vi "Attributes Setup.vi"(11 "IMAQdx Cam in":refnum<class "IMAQdx Cam.lvclass">) -> ()   [LabVIEW 2020, in "IMAQdx Cam.lvclass"]
doc: "The Grab and Attributes Setup example VI allows the user to view the current attributes and settings, update attribute settings, acquire images continuously, and display the images in an image control."
uses:
  IMAQdx Cam.lvclass
  IMAQdx Cam.lvclass/IMAQdx Cam.ctl
panel:
  in  "Filter":string
  in  "error in":errorcluster
  out "Tooltip":string
  out "Units":string
  out "Tab Control Ref":T1
  in  "Tab Control":T2(tab)
  in  "U32 Value Control":u32(slide) scale=4.0..4044.0
  in  "DBL Value Control":dbl(slide) min=17.00000029813964 max=5000000.0 step=1.0 scale=17.00000029813964..5000000.0
  in  "String Value Control":string
  in  "Enum Value Control":u32(ring) items=["Use hardware value", "10-bit", "12-bit", "14-bit", "16-bit"]
  in  "Boolean Value Control":bool=TRUE
  in  "Command Value Control":bool
  in  "Attribute Table":string(tree)="_1"
  in  "stop":bool
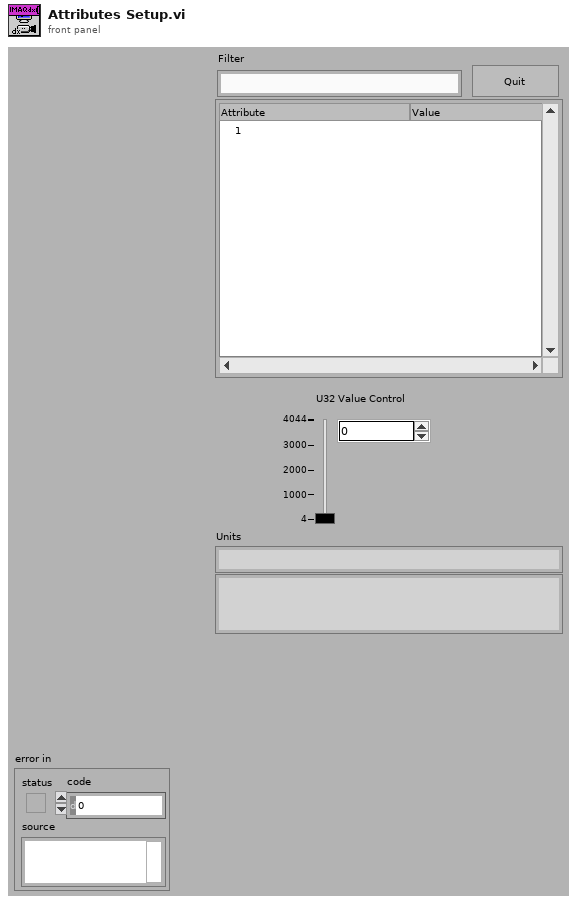
[diagram p1: front panel]
types:
  T1 = cluster{"Tab Control":refnum<vi>, "U32 Value Control":refnum<vi>, "DBL Value Control":refnum<vi>, "String Value Control":refnum<vi>, "Enum Value Control":refnum<vi>, "Boolean Value Control":refnum<vi>, "Command Value Control":refnum<vi>}
  T2 = enum32{"U32", "DBL", "String", "Enum", "Bool", "Command"}
  T3 = typedef "IMAQdx.ctl" = refnum<k21>
  T4 = typedef "eventvkey.ctl" = enum16{"ASCII", "Enter", "Return", "Shift", "Ctrl", "Alt", "Cmd", "Opt", "Caps", "NumLock", "Clear", "Break", "Up", "Down", "Left", "Right", "Insert", "Delete", "Home", "End", "PageUp", "PageDown", "Escape", "Help", "Pause", "ScrollLock", "F1", "F2", "F3", "F4", "F5", "F6", "F7", "F8", "F9", "F10", "F11", "F12", "F13", "F14", "F15", "F16", "F17", "F18", "F19", "F20", "F21", "F22", "F23", "F24", "Play", "VolumeUp", "VolumeDown", "Mute", "Two Byte Char"}
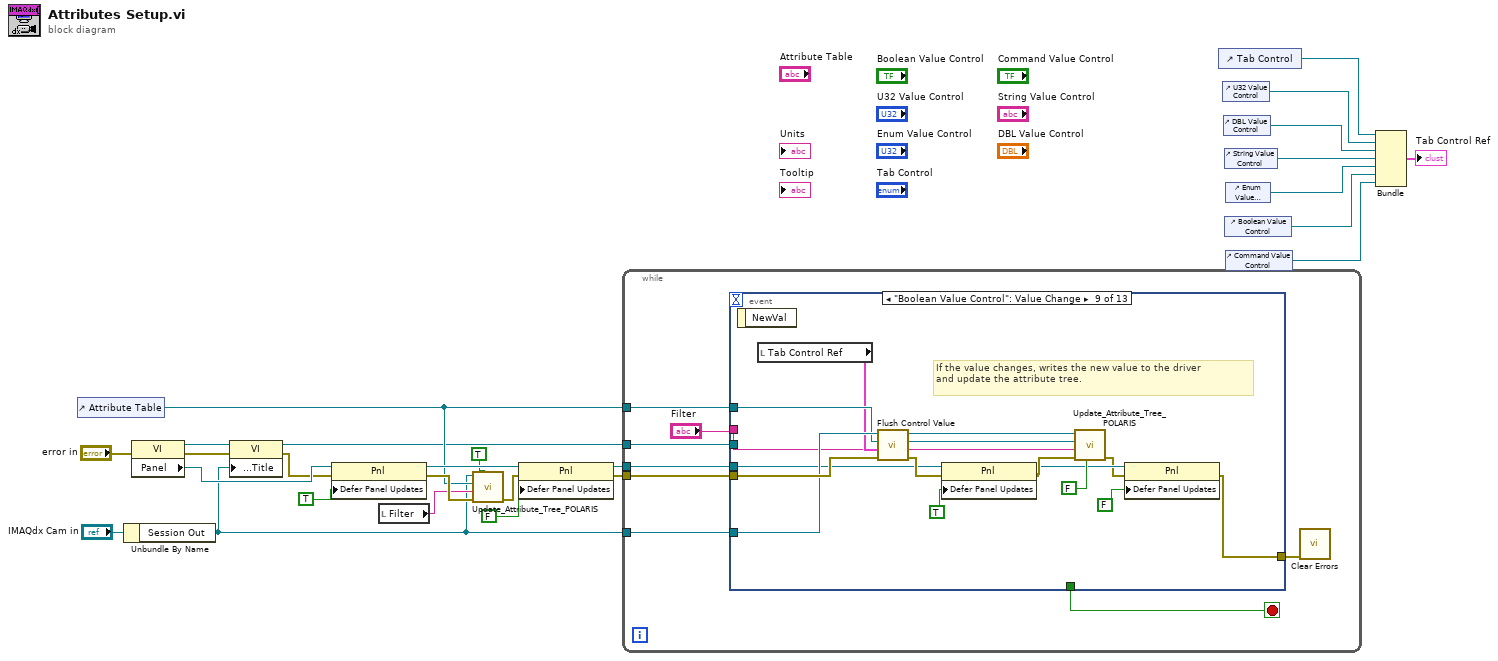
[diagram p0: block diagram]
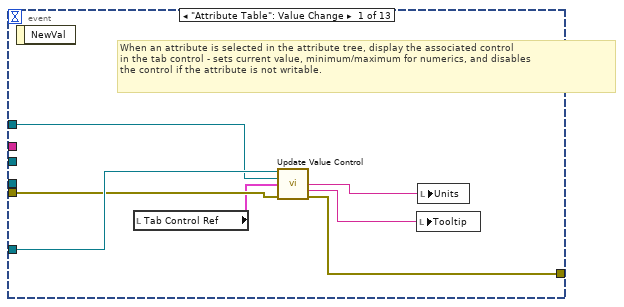
[diagram p2: hidden frame]
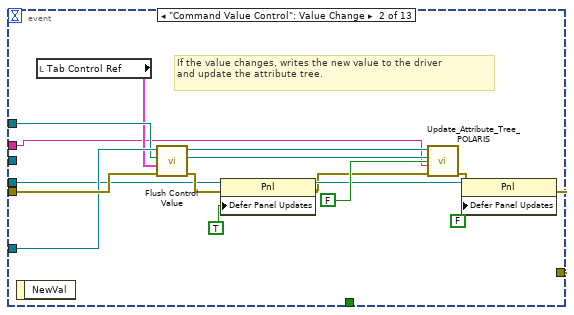
[diagram p3: hidden frame]
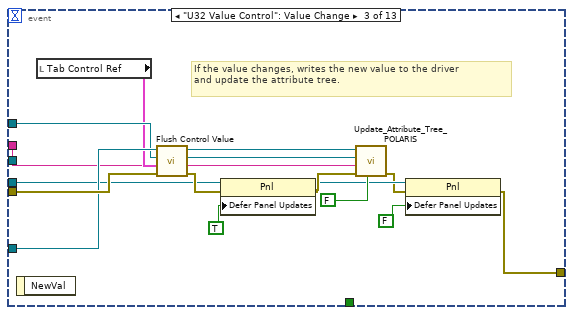
[diagram p4: hidden frame]
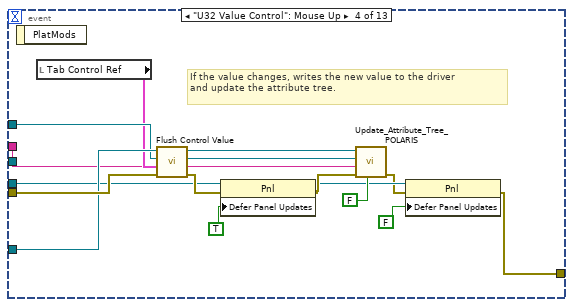
[diagram p5: hidden frame]
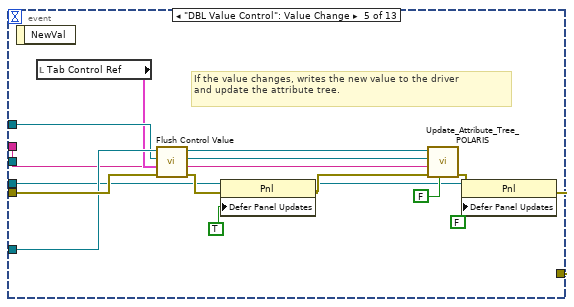
[diagram p6: hidden frame]
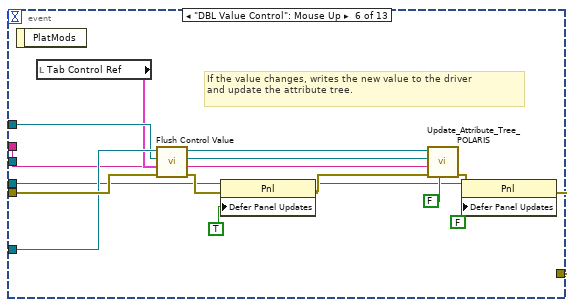
[diagram p7: hidden frame]
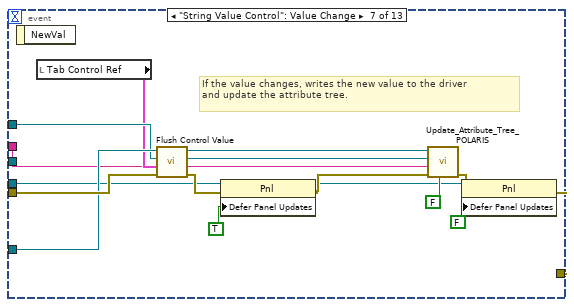
[diagram p8: hidden frame]
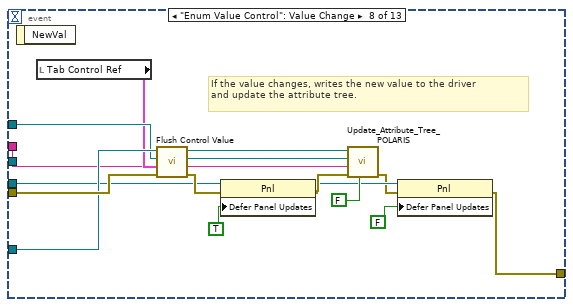
[diagram p9: hidden frame]
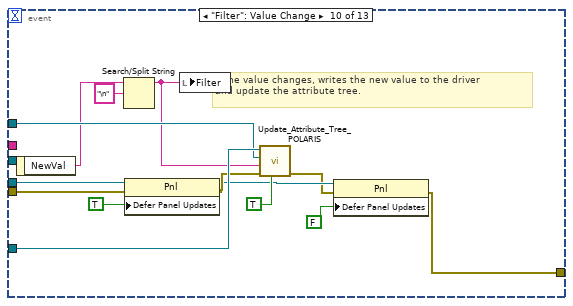
[diagram p10: hidden frame]
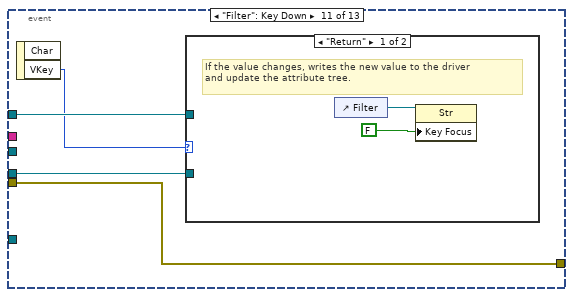
[diagram p11: hidden frame]
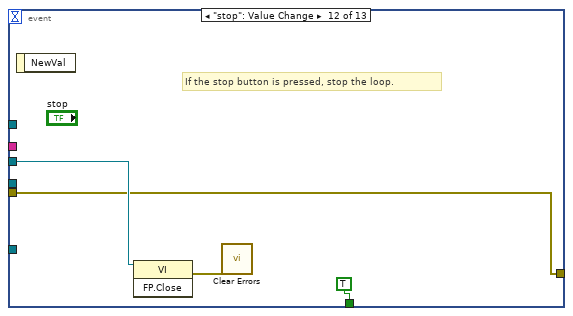
[diagram p13: hidden frame]
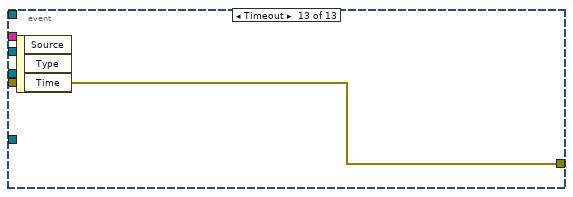
[diagram p14: hidden frame]
diagram:
  n1 = control-ref of="Attribute Table"() -> (w15:refnum<vi>)
  n2 = Unbundle By Name("IMAQdx Cam in") -> ("Session Out"=w6:T3)
  n3 = property class="VI"(error in="error in") -> (reference out=w4:refnum<vi>, error out=w1:errorcluster, "Panel"=w8:refnum<vi>)  [unwired: 1 in]
  n4 = property class="VI"(reference=w4, error in=w1, "Front Panel.Title"=w6) -> (reference out=w3:refnum<vi>, error out=w5:errorcluster)
  n5 = property class="Pnl"(reference=w8, error in=w5, "Defer Panel Updates"=TRUE) -> (reference out=w16:refnum<vi>, error out=w18:errorcluster)
  n6 = local read "Filter"() -> (w10:string)
  n7 = call "Update_Attribute_Tree_POLARIS.vi"("Flush Tree?"=TRUE, "error in"=w18, "Filter"=w10, "Tree Control In"=w15, "Camera Name In"=w6) -> ("error out"=w17:errorcluster)  [unwired: 1 in, 2 out]
  n8 = property class="Pnl"(reference=w16, error in=w17, "Defer Panel Updates"=FALSE ("Flush Tree?")) -> (reference out=w14:refnum<vi>, error out=w11:errorcluster)
  n9 = while {
    tunnel: w11 -> [w33]
    tunnel: w6 -> [w34]
    tunnel: w15 -> [w32]
    tunnel: w14 -> [w31]
    tunnel: w3 -> [w29]
    stop <- w30 stop-if-true
    n10 = event shown="[8] \"Boolean Value Control\": Value Change" {
      selector: _ -> [_ _ _ _ _ _ _ _ _ _ _ _ _]
      dyn-events: _ -> [_ _ _ _ _ _ _ _ _ _ _ _ _]
      timeout: _ -> [_ _ _ _ _ _ _ _ _ _ _ _ _]
      tunnel: w34 -> [w41 w56 w72 w88 w104 w120 w136 w152 w168 w182 _ _ _]
      tunnel: w33 -> [w40 w57 w73 w89 w105 w121 w137 w153 w169 w183 w185 w192 w194]
      tunnel: [w39 w44 w59 w75 w91 w107 w123 w139 w155 w173 w185 w192 w194] -> w27
      tunnel: w32 -> [w35 w54 w70 w86 w102 w118 w134 w150 w166 w181 w187 _ _]
      tunnel: w31 -> [_ w49 w64 w80 w96 w112 w128 w144 w160 w178 w186 _ _]
      tunnel: [_ _ _ _ _ _ _ _ _ _ _ TRUE ("stop") _] -> w30
      tunnel: w29 -> [_ _ _ _ _ _ _ _ _ _ _ w193 _]
      tunnel: "Filter" -> [_ w42 w58 w74 w90 w106 w122 w138 w154 _ _ _ _]
      event "Attribute Table": Value Change {
        # "When an attribute is selected in the attribute tree, display the associated control\nin the tab control - sets current value, minimum/maximum for numerics, and disables\nthe control if the attribute is not writable."
        n11 = event-data() -> ()  [unwired: 2 out]
        n12 = local read "Tab Control Ref"() -> (w38:T1)
        n13 = call "Update Value Control.vi"("Session In"=w41, "Tree Control In"=w35, "Tab Control Ref In"=w38, "error in (no error)"=w40) -> ("Units"=w37:string, "Tooltip"=w36:string, "error out"=w39:errorcluster)  [unwired: 1 in, 8 out]
        n14 = local write "Tooltip"(w36) -> ()
        n15 = local write "Units"(w37) -> ()
      }
      event "Command Value Control": Value Change {
        # "If the value changes, writes the new value to the driver\nand update the attribute tree."
        n16 = event-data() -> ()  [unwired: 2 out]
        n17 = local read "Tab Control Ref"() -> (w53:T1)
        n18 = call "Flush Control Value.vi"("error in (no error)"=w57, "Tab Control Ref In"=w53, "Tree Control In"=w54, "Session In"=w56) -> ("error out"=w50:errorcluster, "Tree Control Out"=w52:refnum<vi>, "Session Out"=w55:T3)  [unwired: 1 out]
        n19 = property class="Pnl"(reference=w49, error in=w50, "Defer Panel Updates"=TRUE) -> (reference out=w47:refnum<vi>, error out=w43:errorcluster)
        n20 = call "Update_Attribute_Tree_POLARIS.vi"("Flush Tree?"=FALSE, "error in"=w43, "Filter"=w42, "Tree Control In"=w52, "Camera Name In"=w55) -> ("error out"=w46:errorcluster)  [unwired: 1 in, 2 out]
        n21 = property class="Pnl"(reference=w47, error in=w46, "Defer Panel Updates"=FALSE) -> (error out=w44:errorcluster)  [unwired: 1 out]
      }
      event "U32 Value Control": Value Change {
        # "If the value changes, writes the new value to the driver\nand update the attribute tree."
        n22 = event-data() -> ()  [unwired: 2 out]
        n23 = local read "Tab Control Ref"() -> (w69:T1)
        n24 = call "Flush Control Value.vi"("error in (no error)"=w73, "Tab Control Ref In"=w69, "Tree Control In"=w70, "Session In"=w72) -> ("error out"=w65:errorcluster, "Tree Control Out"=w68:refnum<vi>, "Session Out"=w71:T3)  [unwired: 1 out]
        n25 = property class="Pnl"(reference=w64, error in=w65, "Defer Panel Updates"=TRUE) -> (reference out=w62:refnum<vi>, error out=w66:errorcluster)
        n26 = call "Update_Attribute_Tree_POLARIS.vi"("Flush Tree?"=FALSE, "error in"=w66, "Filter"=w58, "Tree Control In"=w68, "Camera Name In"=w71) -> ("error out"=w61:errorcluster)  [unwired: 1 in, 2 out]
        n27 = property class="Pnl"(reference=w62, error in=w61, "Defer Panel Updates"=FALSE) -> (error out=w59:errorcluster)  [unwired: 1 out]
      }
      event "U32 Value Control": Mouse Up {
        # "If the value changes, writes the new value to the driver\nand update the attribute tree."
        n28 = event-data() -> ()  [unwired: 2 out]
        n29 = local read "Tab Control Ref"() -> (w85:T1)
        n30 = call "Flush Control Value.vi"("error in (no error)"=w89, "Tab Control Ref In"=w85, "Tree Control In"=w86, "Session In"=w88) -> ("error out"=w81:errorcluster, "Tree Control Out"=w84:refnum<vi>, "Session Out"=w87:T3)  [unwired: 1 out]
        n31 = property class="Pnl"(reference=w80, error in=w81, "Defer Panel Updates"=TRUE) -> (reference out=w78:refnum<vi>, error out=w82:errorcluster)
        n32 = call "Update_Attribute_Tree_POLARIS.vi"("Flush Tree?"=FALSE, "error in"=w82, "Filter"=w74, "Tree Control In"=w84, "Camera Name In"=w87) -> ("error out"=w77:errorcluster)  [unwired: 1 in, 2 out]
        n33 = property class="Pnl"(reference=w78, error in=w77, "Defer Panel Updates"=FALSE) -> (error out=w75:errorcluster)  [unwired: 1 out]
      }
      event "DBL Value Control": Value Change {
        # "If the value changes, writes the new value to the driver\nand update the attribute tree."
        n34 = event-data() -> ()  [unwired: 2 out]
        n35 = local read "Tab Control Ref"() -> (w101:T1)
        n36 = call "Flush Control Value.vi"("error in (no error)"=w105, "Tab Control Ref In"=w101, "Tree Control In"=w102, "Session In"=w104) -> ("error out"=w97:errorcluster, "Tree Control Out"=w100:refnum<vi>, "Session Out"=w103:T3)  [unwired: 1 out]
        n37 = property class="Pnl"(reference=w96, error in=w97, "Defer Panel Updates"=TRUE) -> (reference out=w94:refnum<vi>, error out=w98:errorcluster)
        n38 = call "Update_Attribute_Tree_POLARIS.vi"("Flush Tree?"=FALSE, "error in"=w98, "Filter"=w90, "Tree Control In"=w100, "Camera Name In"=w103) -> ("error out"=w93:errorcluster)  [unwired: 1 in, 2 out]
        n39 = property class="Pnl"(reference=w94, error in=w93, "Defer Panel Updates"=FALSE) -> (error out=w91:errorcluster)  [unwired: 1 out]
      }
      event "DBL Value Control": Mouse Up {
        # "If the value changes, writes the new value to the driver\nand update the attribute tree."
        n40 = event-data() -> ()  [unwired: 2 out]
        n41 = local read "Tab Control Ref"() -> (w117:T1)
        n42 = call "Flush Control Value.vi"("error in (no error)"=w121, "Tab Control Ref In"=w117, "Tree Control In"=w118, "Session In"=w120) -> ("error out"=w113:errorcluster, "Tree Control Out"=w116:refnum<vi>, "Session Out"=w119:T3)  [unwired: 1 out]
        n43 = property class="Pnl"(reference=w112, error in=w113, "Defer Panel Updates"=TRUE) -> (reference out=w110:refnum<vi>, error out=w114:errorcluster)
        n44 = call "Update_Attribute_Tree_POLARIS.vi"("Flush Tree?"=FALSE, "error in"=w114, "Filter"=w106, "Tree Control In"=w116, "Camera Name In"=w119) -> ("error out"=w109:errorcluster)  [unwired: 1 in, 2 out]
        n45 = property class="Pnl"(reference=w110, error in=w109, "Defer Panel Updates"=FALSE) -> (error out=w107:errorcluster)  [unwired: 1 out]
      }
      event "String Value Control": Value Change {
        # "If the value changes, writes the new value to the driver\nand update the attribute tree."
        n46 = event-data() -> ()  [unwired: 2 out]
        n47 = local read "Tab Control Ref"() -> (w133:T1)
        n48 = call "Flush Control Value.vi"("error in (no error)"=w137, "Tab Control Ref In"=w133, "Tree Control In"=w134, "Session In"=w136) -> ("error out"=w129:errorcluster, "Tree Control Out"=w132:refnum<vi>, "Session Out"=w135:T3)  [unwired: 1 out]
        n49 = property class="Pnl"(reference=w128, error in=w129, "Defer Panel Updates"=TRUE) -> (reference out=w126:refnum<vi>, error out=w130:errorcluster)
        n50 = call "Update_Attribute_Tree_POLARIS.vi"("Flush Tree?"=FALSE, "error in"=w130, "Filter"=w122, "Tree Control In"=w132, "Camera Name In"=w135) -> ("error out"=w125:errorcluster)  [unwired: 1 in, 2 out]
        n51 = property class="Pnl"(reference=w126, error in=w125, "Defer Panel Updates"=FALSE) -> (error out=w123:errorcluster)  [unwired: 1 out]
      }
      event "Enum Value Control": Value Change {
        # "If the value changes, writes the new value to the driver\nand update the attribute tree."
        n52 = event-data() -> ()  [unwired: 2 out]
        n53 = local read "Tab Control Ref"() -> (w149:T1)
        n54 = call "Flush Control Value.vi"("error in (no error)"=w153, "Tab Control Ref In"=w149, "Tree Control In"=w150, "Session In"=w152) -> ("error out"=w145:errorcluster, "Tree Control Out"=w148:refnum<vi>, "Session Out"=w151:T3)  [unwired: 1 out]
        n55 = property class="Pnl"(reference=w144, error in=w145, "Defer Panel Updates"=TRUE) -> (reference out=w142:refnum<vi>, error out=w146:errorcluster)
        n56 = call "Update_Attribute_Tree_POLARIS.vi"("Flush Tree?"=FALSE, "error in"=w146, "Filter"=w138, "Tree Control In"=w148, "Camera Name In"=w151) -> ("error out"=w141:errorcluster)  [unwired: 1 in, 2 out]
        n57 = property class="Pnl"(reference=w142, error in=w141, "Defer Panel Updates"=FALSE) -> (error out=w139:errorcluster)  [unwired: 1 out]
      }
      event "Boolean Value Control": Value Change {
        # "If the value changes, writes the new value to the driver\nand update the attribute tree."
        n58 = event-data() -> ()  [unwired: 2 out]
        n59 = local read "Tab Control Ref"() -> (w165:T1)
        n60 = call "Flush Control Value.vi"("error in (no error)"=w169, "Tab Control Ref In"=w165, "Tree Control In"=w166, "Session In"=w168) -> ("error out"=w161:errorcluster, "Tree Control Out"=w164:refnum<vi>, "Session Out"=w167:T3)  [unwired: 1 out]
        n61 = property class="Pnl"(reference=w160, error in=w161, "Defer Panel Updates"=TRUE) -> (reference out=w158:refnum<vi>, error out=w162:errorcluster)
        n62 = call "Update_Attribute_Tree_POLARIS.vi"("Flush Tree?"=FALSE, "error in"=w162, "Filter"=w154, "Tree Control In"=w164, "Camera Name In"=w167) -> ("error out"=w157:errorcluster)  [unwired: 1 in, 2 out]
        n63 = property class="Pnl"(reference=w158, error in=w157, "Defer Panel Updates"=FALSE) -> (error out=w155:errorcluster)  [unwired: 1 out]
      }
      event "Filter": Value Change {
        # "If the value changes, writes the new value to the driver\nand update the attribute tree."
        n64 = event-data() -> ("NewVal"=w172:string)  [unwired: 1 out]
        n65 = Search/Split String(string=w172, search string/char (-)="\n") -> (substring before match=w170:string)  [unwired: 1 in, 2 out]
        n66 = property class="Pnl"(reference=w178, error in=w183, "Defer Panel Updates"=TRUE) -> (reference out=w176:refnum<vi>, error out=w179:errorcluster)
        n67 = local write "Filter"(w170) -> ()
        n68 = call "Update_Attribute_Tree_POLARIS.vi"("Flush Tree?"=TRUE, "error in"=w179, "Filter"=w170, "Tree Control In"=w181, "Camera Name In"=w182) -> ("error out"=w175:errorcluster)  [unwired: 1 in, 2 out]
        n69 = property class="Pnl"(reference=w176, error in=w175, "Defer Panel Updates"=FALSE) -> (error out=w173:errorcluster)  [unwired: 1 out]
      }
      event "Filter": Key Down {
        n70 = event-data() -> ("VKey"=w184:T4)  [unwired: 2 out]
        n71 = case shown="\"Return\"" w184 {
          tunnel: w187 -> [_ _]
          tunnel: w186 -> [_ _]
          frame "Return" {
            # "If the value changes, writes the new value to the driver\nand update the attribute tree."
            n72 = control-ref of="Filter"() -> (w188:refnum<vi>)
            n73 = property class="Str"(reference=w188, "Key Focus"=FALSE) -> ()  [unwired: 1 in, 2 out]
          }
          frame "Enter", Default {
          }
        }
      }
      event "stop": Value Change {
        # "If the stop button is pressed, stop the loop."
        n74 = event-data() -> ()  [unwired: 2 out]
        n75 = invoke class="VI" method="FP.Close"(reference=w193) -> (error out=w191:errorcluster)  [unwired: 2 in, 2 out]
        n76 = call <vilib>:"Clear Errors.vi"("error in (no error)"=w191) -> ()  [unwired: 5 in, 2 out]
      }
      event Timeout {
        n77 = event-data() -> ()  [unwired: 4 out]
      }
    }
    n78 = call <vilib>:"Clear Errors.vi"("error in (no error)"=w27) -> ()  [unwired: 5 in, 2 out]
  }
  n79 = control-ref of="Tab Control"() -> (w26:refnum<vi>)
  n80 = control-ref of="U32 Value Control"() -> (w24:refnum<vi>)
  n81 = control-ref of="DBL Value Control"() -> (w23:refnum<vi>)
  n82 = control-ref of="String Value Control"() -> (w25:refnum<vi>)
  n83 = control-ref of="Boolean Value Control"() -> (w21:refnum<vi>)
  n84 = control-ref of="Enum Value Control"() -> (w22:refnum<vi>)
  n85 = control-ref of="Command Value Control"() -> (w20:refnum<vi>)
  n86 = Bundle("Tab Control"=w26, "U32 Value Control"=w24, "DBL Value Control"=w23, "String Value Control"=w25, "Enum Value Control"=w22, "Boolean Value Control"=w21, "Command Value Control"=w20) -> (→"Tab Control Ref":T1)  [unwired: 1 out]
